vi "Func-엑셀 데이터를 그래프로 출력.vi"() -> ()   [LabVIEW 2015] (continued)
492.03\n492.04\n492.06\n492.08\n492.1\n492.11\n492.13\n492.14\n492.16\n492.18\n492.19\n492.21\n492.23\n492.25\n492.26\n492.28\n492.29\n492.31\n492.33\n492.34\n492.36\n492.38\n492.39\n492.41\n492.43\n492.44\n492.46\n492.48\n492.49\n492.51\n492.53\n492.54\n492.56\n492.58\n492.59\n492.61\n492.63\n492.64\n492.66\n492.68\n492.69\n492.71\n492.73\n492.74\n492.76\n492.78\n492.79\n492.81\n492.83\n492.84\n492.86\n492.88\n492.89\n492.91\n492.93\n492.94\n492.96\n492.98\n492.99\n493.01\n493.03\n493.04\n493.06\n493.08\n493.09\n493.11\n493.13\n493.14\n493.16\n493.18\n493.19\n493.21\n493.23\n493.24\n493.26\n493.28\n493.29\n493.31\n493.33\n493.34\n493.36\n493.38\n493.39\n493.41\n493.43\n493.44\n493.46\n493.48\n493.49\n493.51\n493.53\n493.54\n493.56\n493.58\n493.59\n493.61\n493.63\n493.64\n493.66\n493.68\n493.69\n493.71\n493.73\n493.74\n493.76\n493.78\n493.79\n493.81\n493.83\n493.84\n493.86\n493.88\n493.89\n493.91\n493.93\n493.95\n493.96\n493.98\n493.99\n494.01\n494.03\n494.04\n494.06\n494.08\n494.09\n494.11\n494.13\n494.14\n494.16\n494.18\n494.19\n494.21\n494.23\n494.24\n494.26\n494.28\n494.3\n494.31\n494.33\n494.34\n494.36\n494.38\n494.39\n494.41\n494.43\n494.44\n494.46\n494.48\n494.49\n494.51\n494.53\n494.55\n494.56\n494.58\n494.59\n494.61\n494.63\n494.65\n494.66\n494.68\n494.69\n494.71\n494.73\n494.74\n494.76\n494.78\n494.79\n494.81\n494.83\n494.84\n494.86\n494.88\n494.89\n494.91\n494.93\n494.94\n494.96\n494.98\n494.99\n495.01\n495.03\n495.04\n495.06\n495.08\n495.09\n495.11\n495.13\n495.14\n495.16\n495.18\n495.19\n495.21\n495.23\n495.24\n495.26\n495.28\n495.29\n495.31\n495.33\n495.34\n495.36\n495.38\n495.39\n495.41\n495.43\n495.44\n495.46\n495.48\n495.49\n495.51\n495.53\n495.54\n495.56\n495.58\n495.59\n495.61\n495.63\n495.64\n495.66\n495.68\n495.69\n495.71\n495.73\n495.74\n495.76\n495.78\n495.79\n495.81\n495.83\n495.84\n495.86\n495.88\n495.89\n495.91\n495.93\n495.94\n495.96\n495.98\n495.99\n496.01\n496.03\n496.04\n496.06\n496.08\n496.09\n496.11\n496.13\n496.14\n496.16\n496.18\n496.19\n496.21\n496.23\n496.24\n496.26\n496.28\n496.29\n496.31\n496.33\n496.34\n496.36\n496.38\n496.39\n496.41\n496.43\n496.44\n496.46\n496.48\n496.49\n496.51\n496.53\n496.54\n496.56\n496.58\n496.59\n496.61\n496.63\n496.64\n496.66\n496.68\n496.69\n496.71\n496.73\n496.74\n496.76\n496.78\n496.79\n496.81\n496.83\n496.84\n496.86\n496.88\n496.89\n496.91\n496.93\n496.94\n496.96\n496.98\n496.99\n497.01\n497.03\n497.05\n497.06\n497.08\n497.09\n497.11\n497.13\n497.14\n497.16\n497.18\n497.19\n497.21\n497.23\n497.24\n497.26\n497.28\n497.3\n497.31\n497.33\n497.34\n497.36\n497.38\n497.4\n497.41\n497.43\n497.44\n497.46\n497.48\n497.49\n497.51\n497.53\n497.54\n497.56\n497.58\n497.59\n497.61\n497.63\n497.65\n497.66\n497.68\n497.69\n497.71\n497.73\n497.74\n497.76\n497.78\n497.79\n497.81\n497.83\n497.85\n497.86\n497.88\n497.89\n497.91\n497.93\n497.94\n497.96\n497.98\n498\n498.01\n498.03\n498.04\n498.06\n498.08\n498.09\n498.11\n498.13\n498.14\n498.16\n498.18\n498.19\n498.21\n498.23\n498.24\n498.26\n498.28\n498.29\n498.31\n498.33\n498.34\n498.36\n498.38\n498.39\n498.41\n498.43\n498.45\n498.46\n498.48\n498.5\n498.51\n498.53\n498.54\n498.56\n498.58\n498.59\n498.61\n498.63\n498.64\n498.66\n498.68\n498.69\n498.71\n498.73\n498.74\n498.76\n498.78\n498.79\n498.81\n498.83\n498.84\n498.86\n498.88\n498.89\n498.91\n498.93\n498.94\n498.96\n498.98\n498.99\n499.01\n499.03\n499.04\n499.06\n499.08\n499.09\n499.11\n499.13\n499.14\n499.16\n499.18\n499.19\n499.21\n499.23\n499.24\n499.26\n499.28\n499.29\n499.31\n499.33\n499.34\n499.36\n499.38\n499.39\n499.41\n499.43\n499.44\n499.46\n499.48\n499.49\n499.51\n499.53\n499.54\n499.56\n499.58\n499.59\n499.61\n499.63\n499.64\n499.66\n499.68\n499.69\n499.71\n499.73\n499.74\n499.76\n499.78\n499.8\n499.81\n499.83\n499.84\n499.86\n499.88\n499.89\n499.91\n499.93\n499.94\n499.96\n499.98\n499.99\n500.01\n500.03\n500.04\n500.06\n500.08\n500.09\n500.11\n500.13\n500.15\n500.16\n500.18\n500.19\n500.21\n500.23\n500.24\n500.26\n500.28\n500.29\n500.31\n500.33\n500.34\n500.36\n500.38\n500.4\n500.41\n500.43\n500.44\n500.46\n500.48\n500.5\n500.51\n500.53\n500.54\n500.56\n500.58\n500.59\n500.61\n500.63\n500.64\n500.66\n500.68\n500.69\n500.71\n500.73\n500.75\n500.76\n500.78\n500.79\n500.81\n500.83\n500.85\n500.86\n500.88\n500.89\n500.91\n500.93\n500.94\n500.96\n500.98\n500.99\n501.01\n501.03\n501.04\n501.06\n501.08\n501.1\n501.11\n501.13\n501.14\n501.16\n501.18\n501.19\n501.21\n501.23\n501.24\n501.26\n501.28\n501.29\n501.31\n501.33\n501.34\n501.36\n501.38\n501.39\n501.41\n501.43\n501.44\n501.46\n501.48\n501.49\n501.51\n501.53\n501.54\n501.56\n501.58\n501.59\n501.61\n501.63\n501.64\n501.66\n501.68\n501.69\n501.71\n501.73\n501.74\n501.76\n501.78\n501.8\n501.81\n501.83\n501.84\n501.86\n501.88\n501.89\n501.91\n501.93\n501.94\n501.96\n501.98\n502\n502.01\n502.03\n502.04\n502.06\n502.08\n502.09\n502.11\n502.13\n502.14\n502.16\n502.18\n502.19\n502.21\n502.23\n502.24\n502.26\n502.28\n502.29\n502.31\n502.33\n502.34\n502.36\n502.38\n502.39\n502.41\n502.43\n502.44\n502.46\n502.48\n502.49\n502.51\n502.53\n502.54\n502.56\n502.58\n502.59\n502.61\n502.63\n502.64\n502.66\n502.68\n502.69\n502.71\n502.73\n502.74\n502.76\n502.78\n502.79\n502.81\n502.83\n502.84\n502.86\n502.88\n502.89\n502.91\n502.93\n502.94\n502.96\n502.98\n502.99\n503.01\n503.03\n503.04\n503.06\n503.08\n503.09\n503.11\n503.13\n503.15\n503.16\n503.18\n503.19\n503.21\n503.23\n503.25\n503.26\n503.28\n503.29\n503.31\n503.33\n503.34\n503.36\n503.38\n503.39\n503.41\n503.43\n503.44\n503.46\n503.48\n503.5\n503.51\n503.53\n503.54\n503.56\n503.58\n503.6\n503.61\n503.63\n503.64\n503.66\n503.68\n503.69\n503.71\n503.73\n503.74\n503.76\n503.78\n503.79\n503.81\n503.83\n503.85\n503.86\n503.88\n503.89\n503.91\n503.93\n503.94\n503.96\n503.98\n503.99\n504.01\n504.03\n504.04\n504.06\n504.08\n504.09\n504.11\n504.13\n504.14\n504.16\n504.18\n504.2\n504.21\n504.23\n504.24\n504.26\n504.28\n504.29\n504.31\n504.33\n504.34\n504.36\n504.38\n504.39\n504.41\n504.43\n504.44\n504.46\n504.48\n504.49\n504.51\n504.53\n504.54\n504.56\n504.58\n504.59\n504.61\n504.63\n504.64\n504.66\n504.68\n504.7\n504.71\n504.73\n504.75\n504.76\n504.78\n504.79\n504.81\n504.83\n504.84\n504.86\n504.88\n504.89\n504.91\n504.93\n504.94\n504.96\n504.98\n504.99\n505.01\n505.03\n505.04\n505.06\n505.08\n505.09\n505.11\n505.13\n505.14\n505.16\n505.18\n505.19\n505.21\n505.23\n505.24\n505.26\n505.28\n505.29\n505.31\n505.33\n505.34\n505.36\n505.38\n505.39\n505.41\n505.43\n505.44\n505.46\n505.48\n505.49\n505.51\n505.53\n505.54\n505.56\n505.58\n505.59\n505.61\n505.63\n505.64\n505.66\n505.68\n505.69\n505.71\n505.73\n505.74\n505.76\n505.78\n505.79\n505.81\n505.83\n505.84\n505.86\n505.88\n505.89\n505.91\n505.93\n505.94\n505.96\n505.98\n505.99\n506.01\n506.03\n506.04\n506.06\n506.08\n506.09\n506.11\n506.13\n506.14\n506.16\n506.18\n506.19\n506.21\n506.23\n506.25\n506.26\n506.28\n506.29\n506.31\n506.33\n506.35\n506.36\n506.38\n506.39\n506.41\n506.43\n506.44\n506.46\n506.48\n506.49\n506.51\n506.53\n506.54\n506.56\n506.58\n506.6\n506.61\n506.63\n506.64\n506.66\n506.68\n506.69\n506.71\n506.73\n506.74\n506.76\n506.78\n506.79\n506.81\n506.83\n506.84\n506.86\n506.88\n506.89\n506.91\n506.93\n506.95\n506.96\n506.98\n506.99\n507.01\n507.03\n507.04\n507.06\n507.08\n507.09\n507.11\n507.13\n507.14\n507.16\n507.18\n507.2\n507.21\n507.23\n507.24\n507.26\n507.28\n507.29\n507.31\n507.33\n507.34\n507.36\n507.38\n507.39\n507.41\n507.43\n507.44\n507.46\n507.48\n507.49\n507.51\n507.53\n507.55\n507.56\n507.58\n507.59\n507.61\n507.63\n507.64\n507.66\n507.68\n507.69\n507.71\n507.73\n507.75\n507.76\n507.78\n507.79\n507.81\n507.83\n507.84\n507.86\n507.88\n507.89\n507.91\n507.93\n507.94\n507.96\n507.98\n507.99\n508.01\n508.03\n508.04\n508.06\n508.08\n508.09\n508.11\n508.13\n508.14\n508.16\n508.18\n508.19\n508.21\n508.23\n508.24\n508.26\n508.28\n508.29\n508.31\n508.33\n508.34\n508.36\n508.38\n508.39\n508.41\n508.43\n508.44\n508.46\n508.48\n508.49\n508.51\n508.53\n508.54\n508.56\n508.58\n508.59\n508.61\n508.63\n508.64\n508.66\n508.68\n508.69\n508.71\n508.73\n508.74\n508.76\n508.78\n508.79\n508.81\n508.83\n508.84\n508.86\n508.88\n508.89\n508.91\n508.93\n508.94\n508.96\n508.98\n508.99\n509.01\n509.03\n509.04\n509.06\n509.08\n509.09\n509.11\n509.13\n509.14\n509.16\n509.18\n509.19\n509.21\n509.23\n509.24\n509.26\n509.28\n509.29\n509.31\n509.33\n509.35\n509.36\n509.38\n509.39\n509.41\n509.43\n509.44\n509.46\n509.48\n509.49\n509.51\n509.53\n509.54\n509.56\n509.58\n509.6\n509.61\n509.63\n509.64\n509.66\n509.68\n509.7\n509.71\n509.73\n509.74\n509.76\n509.78\n509.79\n509.81\n509.83\n509.84\n509.86\n509.88\n509.89\n509.91\n509.93\n509.95\n509.96\n509.98\n509.99\n510.01\n510.03\n510.05\n510.06\n510.08\n510.09\n510.11\n510.13\n510.14\n510.16\n510.18\n510.19\n510.21\n510.23\n510.24\n510.26\n510.28\n510.3\n510.31\n510.33\n510.34\n510.36\n510.38\n510.39\n510.41\n510.43\n510.44\n510.46\n510.48\n510.49\n510.51\n510.53\n510.54\n510.56\n510.58\n510.59\n510.61\n510.63\n510.64\n510.66\n510.68\n510.69\n510.71\n510.73\n510.74\n510.76\n510.78\n510.79\n510.81\n510.83\n510.84\n510.86\n510.88\n510.89\n510.91\n510.93\n510.94\n510.96\n510.98\n510.99\n511.01\n511.03\n511.04\n511.06\n511.08\n511.09\n511.11\n511.13\n511.14\n511.16\n511.18\n511.19\n511.21\n511.23\n511.24\n511.26\n511.28\n511.29\n511.31\n511.33\n511.34\n511.36\n511.38\n511.39\n511.41\n511.43\n511.44\n511.46\n511.48\n511.49\n511.51\n511.53\n511.54\n511.56\n511.58\n511.59\n511.61\n511.63\n511.64\n511.66\n511.68\n511.69\n511.71\n511.73\n511.74\n511.76\n511.78\n511.79\n511.81\n511.83\n511.84\n511.86\n511.88\n511.89\n511.91\n511.93\n511.94\n511.96\n511.98\n511.99\n512.01\n512.03\n512.04\n512.06\n512.08\n512.09\n512.11\n512.13\n512.14\n512.16\n512.18\n512.19\n512.21\n512.23\n512.24\n512.26\n512.28\n512.29\n512.31\n512.33\n512.34\n512.36\n512.38\n512.39\n512.41\n512.43\n512.45\n512.46\n512.48\n512.49\n512.51\n512.53\n512.54\n512.56\n512.58\n512.59\n512.61\n512.63\n512.64\n512.66\n512.68\n512.69\n512.71\n512.73\n512.74\n512.76\n512.78\n512.8\n512.81\n512.83\n512.84\n512.86\n512.88\n512.89\n512.91\n512.93\n512.94\n512.96\n512.98\n512.99\n513.01\n513.03\n513.05\n513.06\n513.08\n513.09\n513.11\n513.13\n513.15\n513.16\n513.18\n513.19\n513.21\n513.23\n513.24\n513.26\n513.28\n513.3\n513.31\n513.33\n513.34\n513.36\n513.38\n513.4\n513.41\n513.43\n513.44\n513.46\n513.48\n513.49\n513.51\n513.53\n513.54\n513.56\n513.58\n513.6\n513.61\n513.63\n513.64\n513.66\n513.68\n513.69\n513.71\n513.73\n513.74\n513.76\n513.78\n513.79\n513.81\n513.83\n513.85\n513.86\n513.88\n513.89\n513.91\n513.93\n513.95\n513.96\n513.98\n513.99\n514.01\n514.03\n514.04\n514.06\n514.08\n514.09\n514.11\n514.13\n514.14\n514.16\n514.18\n514.19\n514.21\n514.23\n514.24\n514.26\n514.28\n514.29\n514.31\n514.33\n514.34\n514.36\n514.38\n514.39\n514.41\n514.43\n514.44\n514.46\n514.48\n514.49\n514.51\n514.53\n514.54\n514.56\n514.58\n514.59\n514.61\n514.63\n514.64\n514.66\n514.68\n514.69\n514.71\n514.73\n514.74\n514.76\n514.78\n514.79\n514.81\n514.83\n514.84\n514.86\n514.88\n514.89\n514.91\n514.93\n514.94\n514.96\n514.98\n514.99\n515.01\n515.03\n515.04\n515.06\n515.08\n515.09\n515.11\n515.13\n515.14\n515.16\n515.18\n515.19\n515.21\n515.23\n515.24\n515.26\n515.28\n515.29\n515.31\n515.33\n515.34\n515.36\n515.38\n515.39\n515.41\n515.43\n515.45\n515.46\n515.48\n515.49\n515.51\n515.53\n515.54\n515.56\n515.58\n515.59\n515.61\n515.63\n515.64\n515.66\n515.68\n515.69\n515.71\n515.73\n515.74\n515.76\n515.78\n515.8\n515.81\n515.83\n515.84\n515.86\n515.88\n515.9\n515.91\n515.93\n515.94\n515.96\n515.98\n515.99\n516.01\n516.03\n516.05\n516.06\n516.08\n516.09\n516.11\n516.13\n516.15\n516.16\n516.18\n516.19\n516.21\n516.23\n516.24\n516.26\n516.28\n516.29\n516.31\n516.33\n516.34\n516.36\n516.38\n516.39\n516.41\n516.43\n516.44\n516.46\n516.48\n516.49\n516.51\n516.53\n516.54\n516.56\n516.58\n516.59\n516.61\n516.63\n516.64\n516.66\n516.68\n516.69\n516.71\n516.73\n516.74\n516.76\n516.78\n516.79\n516.81\n516.83\n516.84\n516.86\n516.88\n516.89\n516.91\n516.93\n516.94\n516.96\n516.98\n516.99\n517.01\n517.03\n517.04\n517.06\n517.08\n517.1\n517.11\n517.13\n517.14\n517.16\n517.18\n517.2\n517.21\n517.23\n517.24\n517.26\n517.28\n517.29\n517.31\n517.33\n517.34\n517.36\n517.38\n517.39\n517.41\n517.43\n517.44\n517.46\n517.48\n517.49\n517.51\n517.53\n517.54\n517.56\n517.58\n517.59\n517.61\n517.63\n517.64\n517.66\n517.68\n517.69\n517.71\n517.73\n517.74\n517.76\n517.78\n517.79\n517.81\n517.83\n517.84\n517.86\n517.88\n517.89\n517.91\n517.93\n517.94\n517.96\n517.98\n517.99\n518.01\n518.03\n518.04\n518.06\n518.08\n518.09\n518.11\n518.13\n518.14\n518.16\n518.18\n518.19\n518.21\n518.23\n518.24\n518.26\n518.28\n518.29\n518.31\n518.33\n518.34\n518.36\n518.38\n518.39\n518.41\n518.43\n518.44\n518.46\n518.48\n518.49\n518.51\n518.53\n518.55\n518.56\n518.58\n518.59\n518.61\n518.63\n518.64\n518.66\n518.68\n518.69\n518.71\n518.73\n518.74\n518.76\n518.78\n518.79\n518.81\n518.83\n518.84\n518.86\n518.88\n518.9\n518.91\n518.93\n518.94\n518.96\n518.98\n519\n519.01\n519.03\n519.04\n519.06\n519.08\n519.09\n519.11\n519.13\n519.15\n519.16\n519.18\n519.19\n519.21\n519.23\n519.25\n519.26\n519.28\n519.29\n519.31\n519.33\n519.35\n519.36\n519.38\n519.39\n519.41\n519.43\n519.44\n519.46\n519.48\n519.49\n519.51\n519.53\n519.54\n519.56\n519.58\n519.59\n519.61\n519.63\n519.64\n519.66\n519.68\n519.7\n519.71\n519.73\n519.74\n519.76\n519.78\n519.79\n519.81\n519.83\n519.85\n519.86\n519.88\n519.89\n519.91\n519.93\n519.94\n519.96\n519.98\n519.99\n520.01\n520.03\n520.04\n520.06\n520.08\n520.09\n520.11\n520.13\n520.14\n520.16\n520.18\n520.19\n520.21\n520.23\n520.24\n520.26\n520.28\n520.29\n520.31\n520.33\n520.34\n520.36\n520.38\n520.39\n520.41\n520.43\n520.44\n520.46\n520.48\n520.49\n520.51\n520.53\n520.54\n520.56\n520.58\n520.59\n520.61\n520.63\n520.64\n520.66\n520.68\n520.69\n520.71\n520.73\n520.74\n520.76\n520.78\n520.79\n520.81\n520.83\n520.84\n520.86\n520.88\n520.89\n520.91\n520.93\n520.94\n520.96\n520.98\n520.99\n521.01\n521.03\n521.04\n521.06\n521.08\n521.09\n521.11\n521.13\n521.14\n521.16\n521.18\n521.19\n521.21\n521.23\n521.24\n521.26\n521.28\n521.29\n521.31\n521.33\n521.34\n521.36\n521.38\n521.39\n521.41\n521.43\n521.44\n521.46\n521.48\n521.49\n521.51\n521.53\n521.54\n521.56\n521.58\n521.59\n521.61\n521.63\n521.65\n521.66\n521.68\n521.69\n521.71\n521.73\n521.74\n521.76\n521.78\n521.79\n521.81\n521.83\n521.84\n521.86\n521.88\n521.89\n521.91\n521.93\n521.94\n521.96\n521.98\n522\n522.01\n522.03\n522.04\n522.06\n522.08\n522.09\n522.11\n522.13\n522.14\n522.16\n522.18\n522.19\n522.21\n522.23\n522.25\n522.26\n522.28\n522.29\n522.31\n522.33\n522.35\n522.36\n522.38\n522.39\n522.41\n522.43\n522.45\n522.46\n522.48\n522.49\n522.51\n522.53\n522.54\n522.56\n522.58\n522.6\n522.61\n522.63\n522.64\n522.66\n522.68\n522.69\n522.71\n522.73\n522.74\n522.76\n522.78\n522.79\n522.81\n522.83\n522.84\n522.86\n522.88\n522.89\n522.91\n522.93\n522.94\n522.96\n522.98\n522.99\n523.01\n523.03\n523.05\n523.06\n523.08\n523.09\n523.11\n523.13\n523.15\n523.16\n523.18\n523.19\n523.21\n523.23\n523.24\n523.26\n523.28\n523.29\n523.31\n523.33\n523.34\n523.36\n523.38\n523.39\n523.41\n523.43\n523.44\n523.46\n523.48\n523.49\n523.51\n523.53\n523.54\n523.56\n523.58\n523.59\n523.61\n523.63\n523.64\n523.66\n523.68\n523.69\n523.71\n523.73\n523.74\n523.76\n523.78\n523.79\n523.81\n523.83\n523.84\n523.86\n523.88\n523.89\n523.91\n523.93\n523.94\n523.96\n523.98\n523.99\n524.01\n524.03\n524.04\n524.06\n524.08\n524.09\n524.11\n524.13\n524.14\n524.16\n524.18\n524.19\n524.21\n524.23\n524.24\n524.26\n524.28\n524.29\n524.31\n524.33\n524.34\n524.36\n524.38\n524.39\n524.41\n524.43\n524.44\n524.46\n524.48\n524.49\n524.51\n524.53\n524.54\n524.56\n524.58\n524.59\n524.61\n524.63\n524.64\n524.66\n524.68\n524.69\n524.71\n524.73\n524.75\n524.76\n524.78\n524.79\n524.81\n524.83\n524.84\n524.86\n524.88\n524.89\n524.91\n524.93\n524.94\n524.96\n524.98\n525\n525.01\n525.03\n525.04\n525.06\n525.08\n525.1\n525.11\n525.13\n525.14\n525.16\n525.18\n525.19\n525.21\n525.23\n525.24\n525.26\n525.28\n525.29\n525.31\n525.33\n525.35\n525.36\n525.38\n525.39\n525.41\n525.43\n525.45\n525.46\n525.48\n525.49\n525.51\n525.53\n525.54\n525.56\n525.58\n525.6\n525.61\n525.63\n525.64\n525.66\n525.68\n525.69\n525.71\n525.73\n525.74\n525.76\n525.78\n525.79\n525.81\n525.83\n525.84\n525.86\n525.88\n525.89\n525.91\n525.93\n525.94\n525.96\n525.98\n525.99\n526.01\n526.03\n526.04\n526.06\n526.08\n526.09\n526.11\n526.13\n526.15\n526.16\n526.18\n526.19\n526.21\n526.23\n526.25\n526.26\n526.28\n526.29\n526.31\n526.33\n526.34\n526.36\n526.38\n526.39\n526.41\n526.43\n526.44\n526.46\n526.48\n526.49\n526.51\n526.53\n526.54\n526.56\n526.58\n526.59\n526.61\n526.63\n526.64\n526.66\n526.68\n526.69\n526.71\n526.73\n526.74\n526.76\n526.78\n526.79\n526.81\n526.83\n526.84\n526.86\n526.88\n526.89\n526.91\n526.93\n526.94\n526.96\n526.98\n526.99\n527.01\n527.03\n527.04\n527.06\n527.08\n527.09\n527.11\n527.13\n527.14\n527.16\n527.18\n527.19\n527.21\n527.23\n527.24\n527.26\n527.28\n527.29\n527.31\n527.33\n527.34\n527.36\n527.38\n527.39\n527.41\n527.43\n527.44\n527.46\n527.48\n527.49\n527.51\n527.53\n527.54\n527.56\n527.58\n527.59\n527.61\n527.63\n527.64\n527.66\n527.68\n527.69\n527.71\n527.73\n527.74\n544.54\n544.71\n544.88\n545.05\n545.21\n545.38\n545.55\n545.71\n545.88\n546.05\n546.21\n546.38\n546.55\n546.72\n546.88\n547.05\n547.21\n547.38\n547.55\n547.71\n547.88\n548.05\n548.21\n548.38\n548.55\n548.71\n548.88\n549.05\n549.21\n549.38\n549.55\n549.72\n549.88\n550.05\n550.21\n550.38\n550.55\n550.71\n550.88\n551.05\n551.21\n551.38\n551.55\n551.71\n551.88\n552.05\n552.21\n552.38\n552.55\n552.72\n552.88\n553.05\n553.21\n553.38\n553.55\n553.71\n553.88\n554.05\n554.21\n554.38\n554.55\n554.71\n554.89\n555.06\n555.22\n555.39\n555.56\n555.72\n555.89\n556.06\n556.22\n556.39\n556.56\n556.72\n556.89\n557.06\n557.22\n557.39\n557.56\n557.72\n557.89\n558.06\n558.22\n558.39\n558.56\n558.72\n558.89\n559.06\n559.22\n559.39\n559.56\n559.72\n559.89\n560.06\n560.22\n560.39\n560.56\n560.72\n560.89\n561.06\n561.22\n561.39\n561.56\n561.72\n561.89\n562.06\n562.22\n562.4\n562.56\n562.73\n562.9\n563.06\n563.23\n563.4\n563.56\n563.73\n563.9\n564.07\n564.23\n564.4\n564.57\n564.73\n564.9\n565.06\n565.23\n565.4\n565.56\n565.73\n565.9\n566.06\n566.23\n566.4\n566.56\n566.73\n566.9\n567.06\n567.23\n567.4\n567.56\n567.73\n567.9\n568.06\n568.23\n568.4\n568.57\n568.73\n568.9\n569.07\n569.23\n569.4\n569.55\n569.74\n569.89\n570.06\n570.23\n570.4\n570.56\n570.73\n570.9\n571.06\n571.23\n571.4\n571.56\n571.73\n571.9\n572.06\n572.23\n572.4\n572.56\n572.73\n572.9\n573.07\n573.23\n573.4\n573.56\n573.73\n573.9\n574.07\n574.23\n574.41\n574.57\n574.75\n574.92\n575.08\n575.25\n575.41\n575.58\n575.75\n575.91\n576.08\n576.26\n576.42\n576.59\n576.76\n576.92\n577.09\n577.26\n577.43\n577.6\n577.76\n577.93\n578.1\n578.27\n578.44\n578.61\n578.77\n578.94\n579.11\n579.27\n579.44\n579.62\n579.78\n579.95\n580.11\n580.28\n580.45\n580.61\n580.78\n580.95\n581.12\n581.28\n581.45\n581.61\n581.78\n581.95\n582.11\n582.28\n582.45\n582.62\n582.78\n582.95\n583.11\n583.28\n583.45\n583.61\n583.78\n583.95\n584.11\n584.28\n584.43\n584.44\n584.46\n584.48\n584.49\n584.51\n584.53\n584.54\n584.56\n584.58\n584.59\n584.61\n584.63\n584.64\n584.66\n584.68\n584.69\n584.71\n584.73\n584.74\n584.76\n584.78\n584.79\n584.81\n584.83\n584.84\n584.86\n584.88\n584.89\n584.91\n584.93\n584.94\n584.96\n584.98\n584.99\n585.01\n585.03\n585.04\n585.06\n585.08\n585.09\n585.11\n585.13\n585.14\n585.16\n585.18\n585.19\n585.21\n585.23\n585.24\n585.26\n585.28\n585.29\n585.31\n585.33\n585.34\n585.36\n585.38\n585.39\n585.41\n585.43\n585.44\n585.46\n585.48\n585.49\n585.51\n585.53\n585.54\n585.56\n585.58\n585.59\n585.61\n585.63\n585.64\n585.66\n585.68\n585.69\n585.71\n585.73\n585.74\n585.76\n585.78\n585.79\n585.81\n585.83\n585.84\n585.86\n585.88\n585.9\n585.91\n585.93\n585.94\n585.96\n585.98\n586\n586.01\n586.03\n586.04\n586.06\n586.08\n586.09\n586.11\n586.13\n586.14\n586.16\n586.18\n586.19\n586.21\n586.23\n586.25\n586.26\n586.28\n586.29\n586.31\n586.33\n586.35\n586.36\n586.38\n586.39\n586.41\n586.43\n586.44\n586.46\n586.48\n586.5\n586.51\n
